vi "Initialize Sessions Impl.vi"(6 "initialize and close session behavior":T1, 7 "require single session":bool, 8 "error in":errorcluster, 10 "instrument":refnum<class "ISession Factory.lvclass">, 11 "session reservation in":refnum<class "Session Reservation.lvclass">) -> (0 "error out":errorcluster, 1 "channel lists":string[](array[string]), 2 "sessions":variant[](array[variant]), 3 "session reservation out":refnum<class "Session Reservation.lvclass">, 4 "location unique id":u64, 5 "retry":bool)   [LabVIEW 2020, in "MeasurementLink Session Management.lvlib" / "Session Reservation.lvclass"]
uses:
  Session Reservation.lvclass
  MeasurementLink Instrument/ISession Factory/ISession Factory.lvclass
  Initialize and Close Session Behavior.ctl
  Session Reservation.lvclass/Session Reservation.ctl
  MeasurementLink Instrument/ISession Factory/Session Initialization Parameters.ctl
  MeasurementLink Measurement Server/Helpers/Error Strings Global Internal.vi
  Connection Map/Connection Map.lvclass
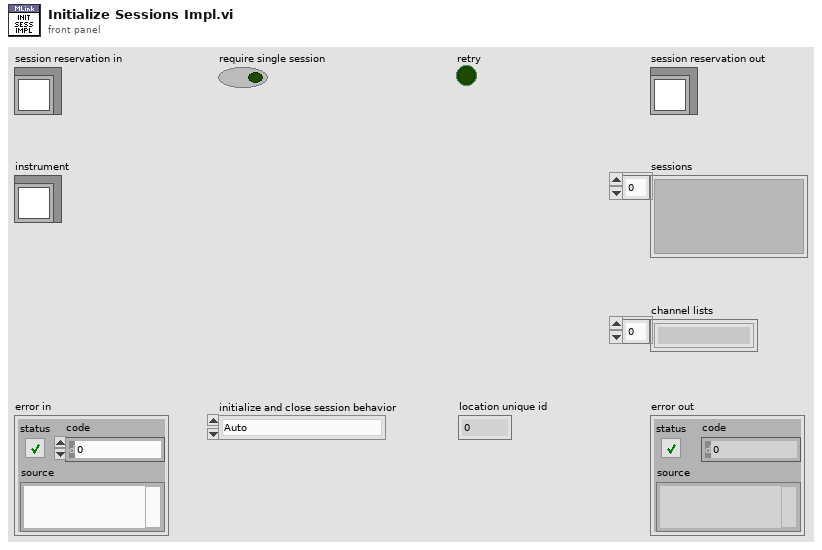
[diagram p1: front panel]
types:
  T1 = typedef "MeasurementLink Session Management.lvlib/Session Reservation.lvclass/Initialize and Close Session Behavior.ctl" = enum16{"Auto", "Initialize and Close", "Attach and Detach", "Initialize and Detach", "Attach and Close"}
  T2 = typedef "MeasurementLink Instrument.lvlib/ISession Factory.lvclass/Session Initialization Parameters.ctl" = cluster{"resource name":string, "session name":string}
  T3 = typedef "MeasurementLink Session Management.lvlib/Session Reservation.lvclass/Data.ctl" = cluster{"session and driver infos":T4[], "pin or relay names":string[], "connection map":refnum<class "Connection Map.lvclass">, "pin map context":T9, "reservation observer":refnum<class "IReservationObserver.lvclass">, "dvr valid":bool}
  T4 = typedef "MeasurementLink Session Management.lvlib/Session Reservation.lvclass/Session and Driver Info.ctl" = cluster{"session info":T5, "session":variant, "session factory":refnum<class "ISession Factory.lvclass">, "initialize and close session behavior":T8}
  T5 = typedef "MeasurementLink Session Management Client.lvlib/ni_measurementlink_sessionmanagement_v1_SessionInformation.ctl" = cluster{"session":T6, "resource_name":string, "channel_list":string, "instrument_type_id":string, "session_exists":bool, "channel_mappings":T7[]}
  T6 = typedef "MeasurementLink Session Management Client.lvlib/nidevice_grpc_Session.ctl" = cluster{"name":string}
  T7 = typedef "MeasurementLink Session Management Client.lvlib/ni_measurementlink_sessionmanagement_v1_ChannelMapping.ctl" = cluster{"pin_or_relay_name":string, "site":i32, "channel":string}
  T8 = typedef "MeasurementLink Instrument.lvlib/ISession Factory.lvclass/Initialize and Close Session Behavior.ctl" = enum16{"Initialize and Close", "Attach and Detach", "Initialize and Detach", "Attach and Close"}
  T9 = typedef "MeasurementLink Session Management Client.lvlib/ni_measurementlink_PinMapContext.ctl" = cluster{"pin_map_id":string, "sites":i32[]}
  T10 = typedef "MeasurementLink Instrument.lvlib/ISession Factory.lvclass/Remote Connection Options.ctl" = cluster{"session name":string, "address":string, "port":u32}
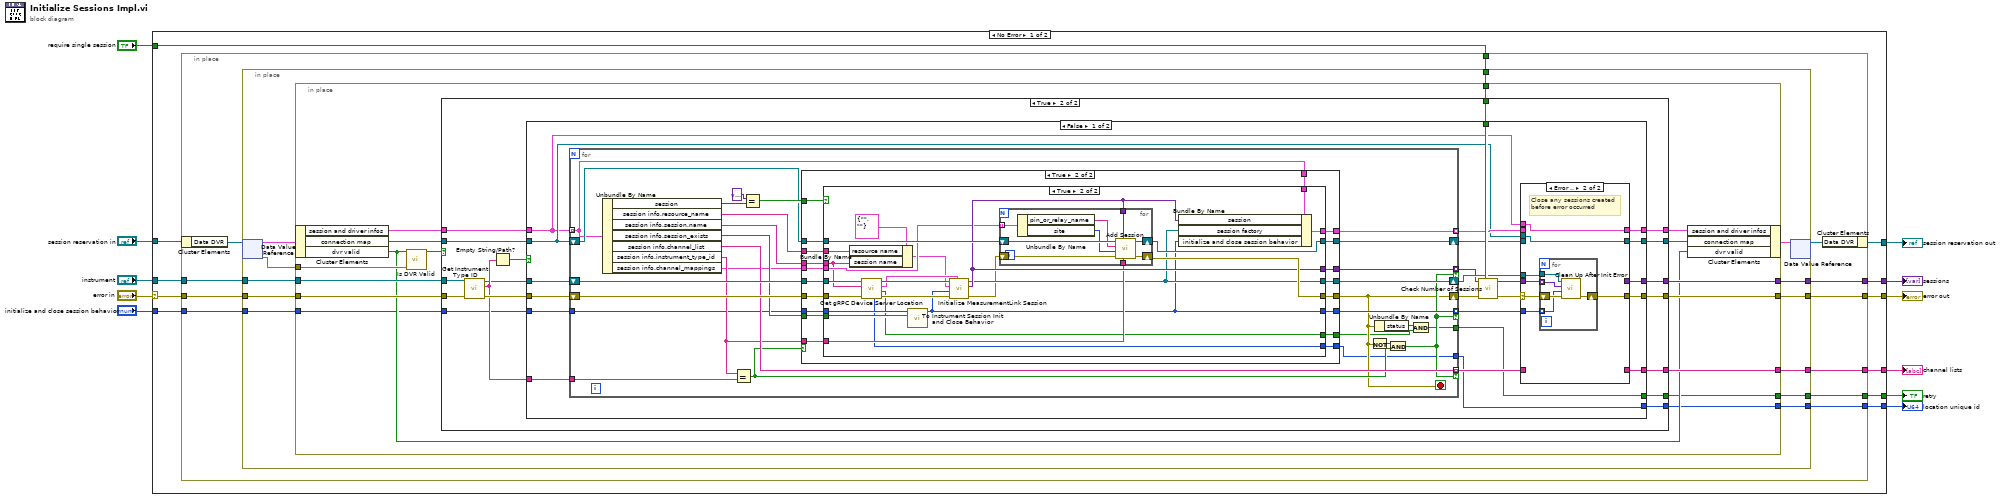
[diagram p0: block diagram]
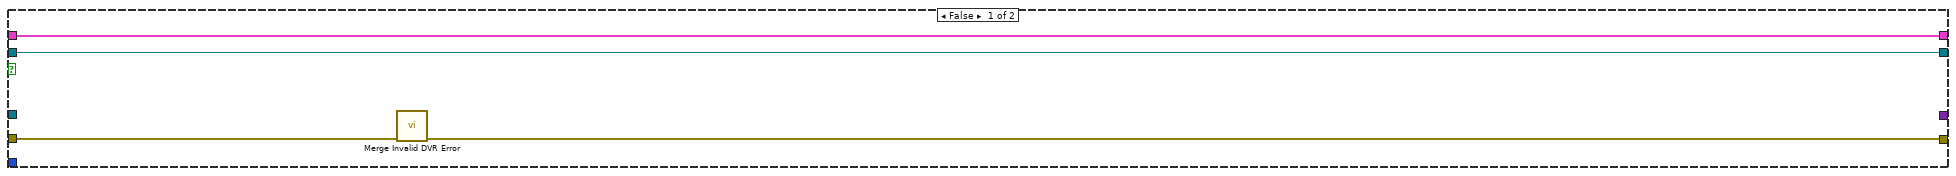
[diagram p2: hidden frame]
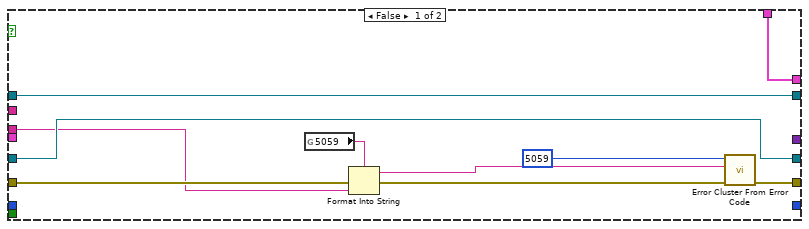
[diagram p5: hidden frame]
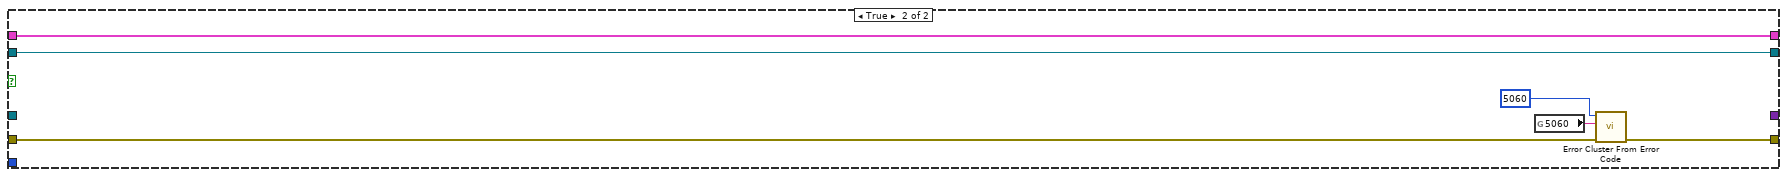
[diagram p6: hidden frame]
diagram:
  n1 = case shown="No Error" "error in" {
    selector: "error in" -> [w19 w224]
    tunnel: "session reservation in" -> [w16 w223]
    tunnel: "instrument" -> [w18 _]
    tunnel: [w22 _] -> w9
    tunnel: [w21 w224] -> w8
    tunnel: [w20 _] -> w7
    tunnel: [w15 w223] -> w4
    tunnel: "require single session" -> [w17 _]
    tunnel: "initialize and close session behavior" -> [w14 _]
    tunnel: [w13 _] -> w2
    tunnel: [w12 _] -> w1
    frame No Error {
      n2 = in-place {
        in-place-border: [w33] -> w22
        in-place-border: [w32] -> w21
        in-place-border: [w31] -> w20
        in-place-border: w19 -> [w30]
        in-place-border: w18 -> [w29]
        in-place-border: w17 -> [w28]
        in-place-border: w14 -> [w25]
        in-place-border: [w24] -> w13
        in-place-border: [w23] -> w12
        n3 = in-place-cluster #1(w16) -> ("Data DVR"=w27:refnum<data-value>)
        n4 = in-place {
          in-place-border: [w45] -> w33
          in-place-border: [w44] -> w32
          in-place-border: [w43] -> w31
          in-place-border: w30 -> [w42]
          in-place-border: w29 -> [w41]
          in-place-border: w28 -> [w40]
          in-place-border: w25 -> [w36]
          in-place-border: [w35] -> w24
          in-place-border: [w34] -> w23
          n5 = in-place-dvr #2(w27) -> (w39:T3, w38:errorcluster)
          n6 = in-place {
            in-place-border: [w61] -> w45
            in-place-border: [w60] -> w44
            in-place-border: [w59] -> w43
            in-place-border: w42 -> [w51]
            in-place-border: w41 -> [w50]
            in-place-border: w40 -> [w58]
            in-place-border: w38 -> [w54]
            in-place-border: w36 -> [w48]
            in-place-border: [w47] -> w35
            in-place-border: [w46] -> w34
            n7 = in-place-cluster #3(w39) -> ("session and driver infos"=w57:T4[], "connection map"=w56:refnum<class "Connection Map.lvclass">, "dvr valid"=w49:bool)
            n8 = call "Is DVR Valid.vi"("dvr error in"=w54, "dvr valid"=w49) -> ("dvr valid"=w53:bool)  [unwired: 9 in]
            n9 = case shown="True" w53 {
              tunnel: [_ w82] -> w61
              tunnel: [w62 w81] -> w60
              tunnel: [_ w80] -> w59
              tunnel: w58 -> [_ w79]
              tunnel: [w64 w78] -> w52
              tunnel: w57 -> [w64 w77]
              tunnel: w56 -> [w65 w76]
              tunnel: [w65 w75] -> w55
              tunnel: w51 -> [w63 w74]
              tunnel: w50 -> [_ w73]
              tunnel: w48 -> [_ w68]
              tunnel: [_ w67] -> w47
              tunnel: [_ w66] -> w46
              frame False {
                n10 = call "Merge Invalid DVR Error.vi"("error in (no error)"=w63) -> ("error out"=w62:errorcluster)  [unwired: 10 in]
              }
              frame True {
                n11 = call-dynamic "Get Instrument Type ID.vi"("error in (no error)"=w74, "session factory in"=w73) -> ("error out"=w72:errorcluster, "instrument type id"=w71:string, "session factory out"=w70:refnum<class "ISession Factory.lvclass">)  [unwired: 7 in]
                n12 = Empty String/Path?(string/path=w71) -> (empty?=w69:bool)
                n13 = case shown="False" w69 {
                  tunnel: w77 -> [w87 w222]
                  tunnel: [w105 _] -> w82
                  tunnel: [w104 w219] -> w81
                  tunnel: [w103 _] -> w80
                  tunnel: [w89 w222] -> w78
                  tunnel: w71 -> [w102 _]
                  tunnel: w70 -> [w101 _]
                  tunnel: w72 -> [w100 w218]
                  tunnel: w79 -> [w99 _]
                  tunnel: w76 -> [w90 w217]
                  tunnel: [w88 w217] -> w75
                  tunnel: w68 -> [w86 _]
                  tunnel: [w84 _] -> w67
                  tunnel: [w83 _] -> w66
                  frame False {
                    n14 = for {
                      tunnel: w87 -> [w134] mode=indexing
                      tunnel: [w149] -> w93 mode=indexing if=w128
                      shift-right: [w127] -> w95
                      shift-left: w100 -> [w145]
                      tunnel: [w143] -> w97 mode=indexing if=w128
                      tunnel: [w148] -> w98 mode=indexing
                      tunnel: w102 -> [w147]
                      shift-right: [w136] -> w96
                      shift-left: w101 -> [w146]
                      shift-right: [w133] -> w91
                      shift-left: w90 -> [w135]
                      tunnel: w86 -> [w130]
                      tunnel: [w129] -> w85 mode=indexing if=w128
                      tunnel: [w125] -> w84
                      tunnel: [w123] -> w83
                      stop <- w127 stop-if-true
                      n15 = Unbundle By Name(w134) -> ("session"=w142:variant, "session info.resource_name"=w144:string, "session info.session.name"=w150:string, "session info.session_exists"=w137:bool, "session info.channel_list"=w143:string, "session info.instrument_type_id"=w132:string, "session info.channel_mappings"=w131:T7[])
                      n16 = Equal?(x=w132, y=w147) -> (x = y?=w138:bool)
                      n17 = Equal?(x=variant, y=w142) -> (x = y?=w141:bool)
                      n18 = case shown="True" w138 {
                        tunnel: w150 -> [_ w173]
                        tunnel: [_ w169] -> w149
                        tunnel: w144 -> [_ w172]
                        tunnel: w137 -> [_ w171]
                        tunnel: [w153 w170] -> w127
                        tunnel: w134 -> [w154 w168]
                        tunnel: [w154 w167] -> w148
                        tunnel: w146 -> [w152 w166]
                        tunnel: w145 -> [w153 w165]
                        tunnel: w141 -> [_ w164]
                        tunnel: [w152 w163] -> w136
                        tunnel: w135 -> [w151 w162]
                        tunnel: [w151 w161] -> w133
                        tunnel: w132 -> [_ w160]
                        tunnel: w131 -> [_ w159]
                        tunnel: w130 -> [_ w158]
                        tunnel: [_ w157] -> w129
                        tunnel: [_ w156] -> w124
                        tunnel: [_ w155] -> w123
                        frame False {
                        }
                        frame True {
                          n19 = case shown="True" w164 {
                            tunnel: w173 -> [w175 w189]
                            tunnel: w172 -> [_ w190]
                            tunnel: w171 -> [_ w193]
                            tunnel: [w182 w199] -> w170
                            tunnel: [_ w198] -> w169
                            tunnel: w168 -> [w181 w207]
                            tunnel: [w181 w206] -> w167
                            tunnel: w166 -> [w176 w205]
                            tunnel: w165 -> [w180 w186]
                            tunnel: [w176 w195] -> w163
                            tunnel: w162 -> [w174 w201]
                            tunnel: [w174 w200] -> w161
                            tunnel: w160 -> [_ w197]
                            tunnel: w159 -> [_ w196]
                            tunnel: w158 -> [_ w194]
                            tunnel: [_ w192] -> w157
                            tunnel: [_ w185] -> w156
                            tunnel: [_ w184] -> w155
                            frame False {
                              n20 = global read "Error Strings Global Internal.vi" "5059"() -> (w177:string)
                              n21 = Format Into String(format string=w177, error in=w180, w175) -> (resulting string=w178:string, error out=w179:errorcluster)  [unwired: 1 in]
                              n22 = call <vilib>:"Error Cluster From Error Code.vi"("error in (no error)"=w179, "error message (\"\")"=w178, "error code (0)"=5059) -> ("error out"=w182:errorcluster)  [unwired: 6 in]
                            }
                            frame True {
                              n23 = Bundle By Name(cluster=T2 {"resource name"="", "session name"=""} ("session initialization details"), "resource name"=w190, "session name"=w189) -> (w188:T2)
                              n24 = call "Get gRPC Device Server Location.vi"("error in"=w186, "session name"=w189, "instrument in"=w205) -> ("error out"=w203:errorcluster, "using device service"=w185:bool, "remote connection options"=w202:T10, "instrument out"=w204:refnum<class "ISession Factory.lvclass">, "location unique id"=w184:u64)  [unwired: 4 in]
                              n25 = call "To Instrument Session Init and Close Behavior.vi"("session exists"=w193, "initialize and close session behavior"=w194) -> ("instrument initialize and close session behavior"=w192:T8)  [unwired: 9 in]
                              n26 = call-dynamic "Initialize MeasurementLink Session.vi"("remote connection options"=w202, "error in (no error)"=w203, "initialize and close session behavior"=w192, "session initialization parameters"=w188, "session factory in"=w204) -> ("error out"=w187:errorcluster, "session out"=w198:variant, "session factory out"=w195:refnum<class "ISession Factory.lvclass">)  [unwired: 4 in]
                              n27 = for {
                                tunnel: w198 -> [w212]
                                tunnel: w197 -> [w211]
                                shift-right: [w215] -> w200
                                shift-left: w201 -> [w216]
                                shift-right: [w213] -> w199
                                shift-left: w187 -> [w214]
                                tunnel: w196 -> [w210] mode=indexing
                                n28 = Unbundle By Name(w210) -> ("pin_or_relay_name"=w209:string, "site"=w208:i32)
                                n29 = call "Add Session.vi"("instrument type id"=w211, "session to add"=w212, "error in"=w214, "site"=w208, "pin or relay name"=w209, "connection map in"=w216) -> ("error out"=w213:errorcluster, "connection map out"=w215:refnum<class "Connection Map.lvclass">)  [unwired: 4 in]
                              }
                              n30 = Bundle By Name(cluster=w207, "session"=w198, "session factory"=w195, "initialize and close session behavior"=w192) -> (w206:T4)
                            }
                          }
                        }
                      }
                      n31 = Not(x=w127) -> (.not. x?=w139:bool)
                      n32 = Unbundle By Name(w127) -> ("status"=w126:bool)
                      n33 = And(x=w139, y=w138) -> (x .and. y?=w128:bool)
                      n34 = And(x=w126, y=w124) -> (x .and. y?=w125:bool)
                    }
                    n35 = call "Check Number of Sessions.vi"("require single session"=w99, "error in"=w95, "sessions in"=w93) -> ("error out"=w94:errorcluster, "sessions out"=w92:variant[])  [unwired: 7 in]
                    n36 = case shown="Error .." w94 {
                      selector: w94 -> [w110 w113]
                      tunnel: [w110 w116] -> w104
                      tunnel: w92 -> [w109 w114]
                      tunnel: [w109 _] -> w105
                      tunnel: w98 -> [w108 _]
                      tunnel: [w108 w117] -> w89
                      tunnel: w97 -> [w107 _]
                      tunnel: [w107 _] -> w103
                      tunnel: w87 -> [_ w117]
                      tunnel: w96 -> [_ w115]
                      tunnel: w91 -> [w106 _]
                      tunnel: [w106 w112] -> w88
                      tunnel: w90 -> [_ w112]
                      tunnel: w85 -> [_ w111]
                      frame No Error {
                      }
                      frame Error {
                        # "Close any sessions created\nbefore error occurred"
                        n37 = for {
                          tunnel: w115 -> [w121]
                          tunnel: w114 -> [w120] mode=indexing
                          shift-right: [w122] -> w116
                          shift-left: w113 -> [w119]
                          tunnel: w111 -> [w118] mode=indexing
                          n38 = call-dynamic "Clean Up After Init Error.vi"("error in"=w119, "initialize and close session behavior"=w118, "session in"=w120, "session factory in"=w121) -> ("error out"=w122:errorcluster)  [unwired: 7 in]
                        }
                      }
                    }
                  }
                  frame True {
                    n39 = global read "Error Strings Global Internal.vi" "5060"() -> (w220:string)
                    n40 = call <vilib>:"Error Cluster From Error Code.vi"("error in (no error)"=w218, "error message (\"\")"=w220, "error code (0)"=5060) -> ("error out"=w219:errorcluster)  [unwired: 6 in]
                  }
                }
              }
            }
            n41 = in-place-cluster #3("session and driver infos"=w52, "connection map"=w55, "dvr valid"=w49) -> (w37:T3)
          }
          n42 = in-place-dvr #2(w37) -> (w26:refnum<data-value>)  [unwired: 1 out]
        }
        n43 = in-place-cluster #1("Data DVR"=w26) -> (w15:refnum<class "Session Reservation.lvclass">)
      }
    }
    frame Error {
    }
  }
  "error out" <- w8
  "sessions" <- w9
  "channel lists" <- w7
  "session reservation out" <- w4
  "retry" <- w2
  "location unique id" <- w1
